vi "Polymorphic.vi"   [LabVIEW 2017, in "G#MethodTemplates.lvclass"]
uses:
  G#MethodTemplates.lvclass
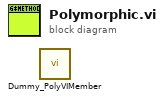
[diagram p0: block diagram]
diagram:
  n1 = call "Dummy_PolyVIMember.vi"() -> ()  [unwired: 20 in]
